vi "Wrapper.vi"(0 "measurement configuration":T1={"Vin SMU Channel"="Lorem ipsum dolor sit", "Range"=1.2, "Resolution in Digits"=0.0, "Voltage Config Str"="", "Current Config Str"="", "Vin SMU Pin"="", "Device Name Pin"=""} {"Resolution in Digits" items=["3 1/2"=3.5, "4 1/2"=4.5, "5 1/2"=5.5, "6 1/2"=6.5, "7 1/2"=7.5]}, 5 "Vin SMU":refnum<k15>="Dev1", 7 "Device Name":refnum<k15>="Dev1", 11 "error in":errorcluster) -> (4 "measurement results":T3={"Measurement "=0.0, "Signal Out of Range"=FALSE, "Measurement from SMU Str"="Empty", "Waveform Graph"=[0.0]} {"Measurement" format="%.6p"}, 15 "error out":errorcluster)   [LabVIEW 2021, in "Voltage Measurement.lvlib"]
uses:
  Voltage Measurement.lvlib
  Measurement Results.ctl
  Measurement Configuration.ctl
  <instrlib>/niDMM/nidmm.llb/niDMM Resolution in Digits.ctl
  MeasurementCore/controls/Voltage Config.ctl
  MeasurementCore/controls/Current Config.ctl
  8052c3e2-2d3c-4b5d-8ebd-80e283c36217.vi
  89afc385-0980-489f-8757-53e797cfab6b.vi
  4d43a4d9-7ba6-4b96-af49-ff976aab273c.vi
  8052c3e2-2d3c-4b5d-8ebd-80e283c36217.vi/6651a77e-856e-4bcd-af5a-c0c13b264cc1.vi
  89afc385-0980-489f-8757-53e797cfab6b.vi/6651a77e-856e-4bcd-af5a-c0c13b264cc1.vi
  4d43a4d9-7ba6-4b96-af49-ff976aab273c.vi/331b549c-fcf8-43d9-8a1e-5b3c0091a99c.vi
  <vilib>/JDP Science/JSONtext/JSON text to Variant.vi
  <vilib>/JDP Science/JSONtext/Variant to JSON Text.vi
  <vilib>/JDP Science/JSONtext/LVClass Serializer/JSONtext LVClass Serializer.lvclass
  MeasurementCore/Main_Voltage Measurement.lvlib
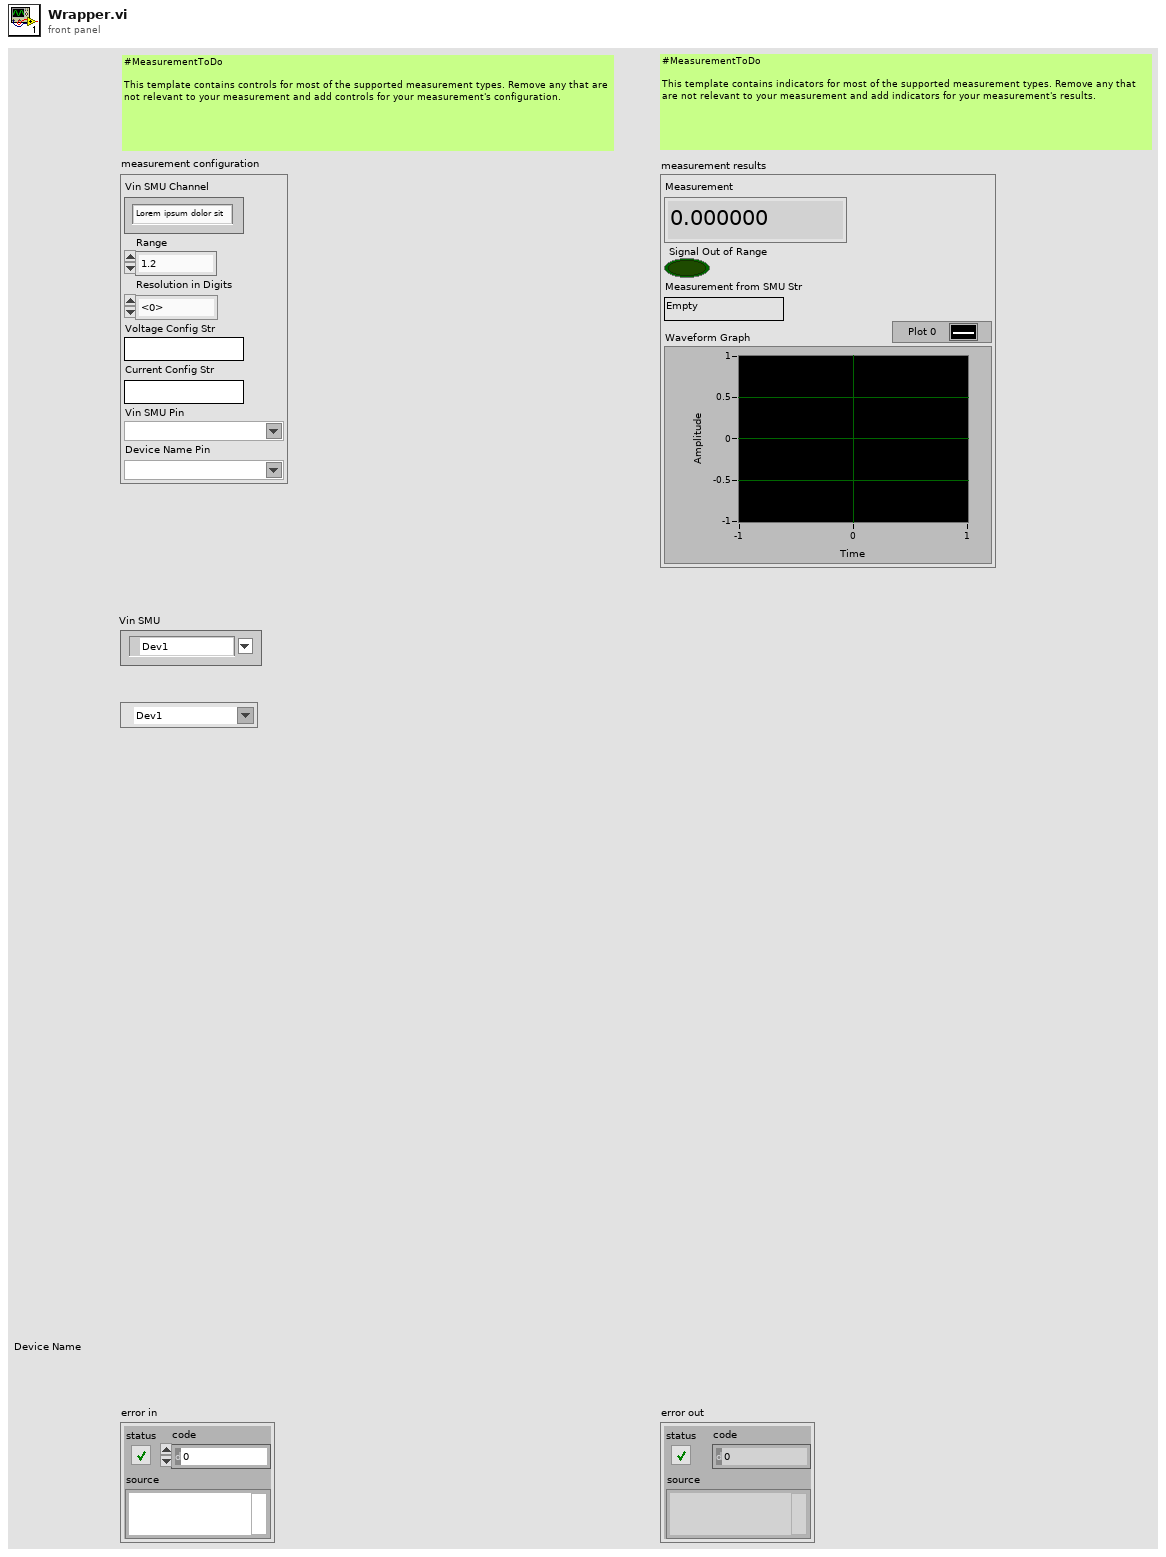
[diagram p1: front panel]
types:
  T1 = typedef "Voltage Measurement.lvlib/Measurement Configuration.ctl" = cluster{"Vin SMU Channel":string, "Range":dbl, "Resolution in Digits":T2, "Voltage Config Str":string, "Current Config Str":string, "Vin SMU Pin":string, "Device Name Pin":string}
  T2 = typedef "niDMM Resolution in Digits.ctl" = dbl
  T3 = typedef "Voltage Measurement.lvlib/Measurement Results.ctl" = cluster{"Measurement ":dbl, "Signal Out of Range":bool, "Measurement from SMU Str":string, "Waveform Graph":dbl[]}
  T4 = typedef "Main_Voltage Measurement.lvlib/Current Config.ctl" = cluster{"Current Limit":dbl, "Current Limit Range":dbl}
  T5 = typedef "Main_Voltage Measurement.lvlib/Voltage Config.ctl" = cluster{"Voltage Level":dbl, "Voltage Level Range":dbl}
  T6 = typedef "Main_Voltage Measurement.lvlib/Measurement.ctl" = cluster{"Voltage Measurement":dbl, "Current Measurement":dbl}
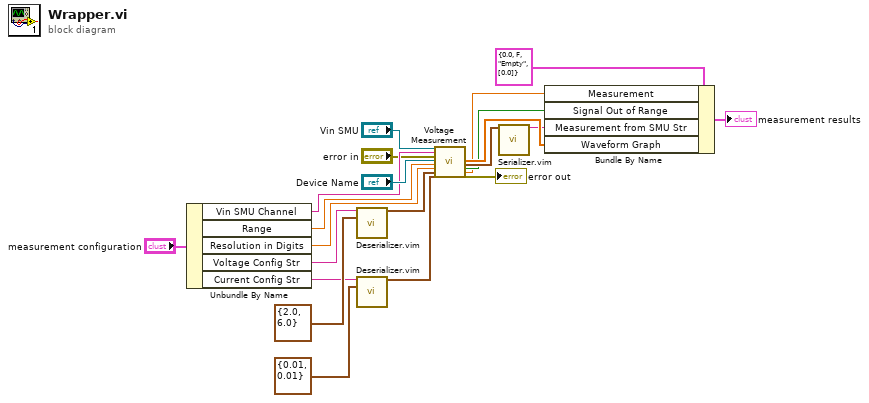
[diagram p0: block diagram]
diagram:
  n1 = Unbundle By Name("measurement configuration") -> ("Vin SMU Channel"=w11:string, "Range"=w10:dbl, "Resolution in Digits"=w9:T2, "Voltage Config Str"=w6:string, "Current Config Str"=w3:string)
  n2 = call "Deserializer.vim"("Flattened Data"=w6, "Data Type"=T5 {"Voltage Level"=2.0, "Voltage Level Range"=6.0} ("Voltage Config")) -> ("Data Out"=w5:T5)  [unwired: 12 in, 1 out]
  n3 = call "Deserializer.vim"("Flattened Data"=w3, "Data Type"=T4 {"Current Limit"=0.01, "Current Limit Range"=0.01} ("Current Config")) -> ("Data Out"=w2:T4)  [unwired: 12 in, 1 out]
  n4 = call "Voltage Measurement.vi"("Vin SMU"="Vin SMU", "Vin SMU Channel"=w11, "error in"="error in", "Device Name"="Device Name", "Range"=w10, "Resolution in Digits"=w9, "Voltage Config"=w5, "Current Config"=w2) -> ("Waveform Graph"=w19:dbl[], "Measurement from SMU"=w18:T6, "Signal Out of Range"=w16:bool, "Measurement"=w15:dbl, "error out"=→"error out":errorcluster)  [unwired: 15 in]
  n5 = call "Serializer.vim"("Anything"=w18) -> ("Flattened Data"=w17:string)  [unwired: 13 in, 1 out]
  n6 = Bundle By Name(cluster=T3 {"Measurement "=0.0, "Signal Out of Range"=FALSE, "Measurement from SMU Str"="Empty", "Waveform Graph"=[0.0]} ("measurement results"), "Measurement"=w15, "Signal Out of Range"=w16, "Measurement from SMU Str"=w17, "Waveform Graph"=w19) -> (→"measurement results":T3)
